vi "Calibration Routine(SubVI).vi"(10 "Calibrate":bool, 11 "File Path (Image Calibration 1)":path=path "\\\\hs2.lboro.ac.uk\\mmbc4/1_Univesity Work/Mechatronics/Machine Vision/Harry_Kane_Project/A3_table_cal_2.png") -> (0 "error out":errorcluster, 1 "Boolean":bool, 3 "Refnum out":T1(plugin-control))   [LabVIEW 2013]
uses:
  <vilib>/vision/driver/NI_Vision_Acquisition_Software.lvlib
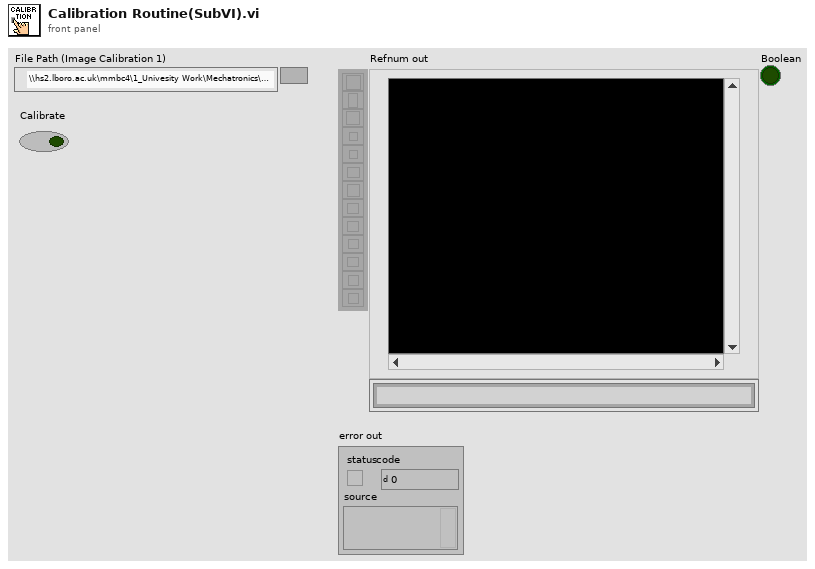
[diagram p1: front panel]
types:
  T1 = typedef "IMAQ Image.ctl" = refnum<image>
  T2 = typedef "Image Type" = u32
  T3 = typedef "IMAQdx.ctl" = refnum<k21>
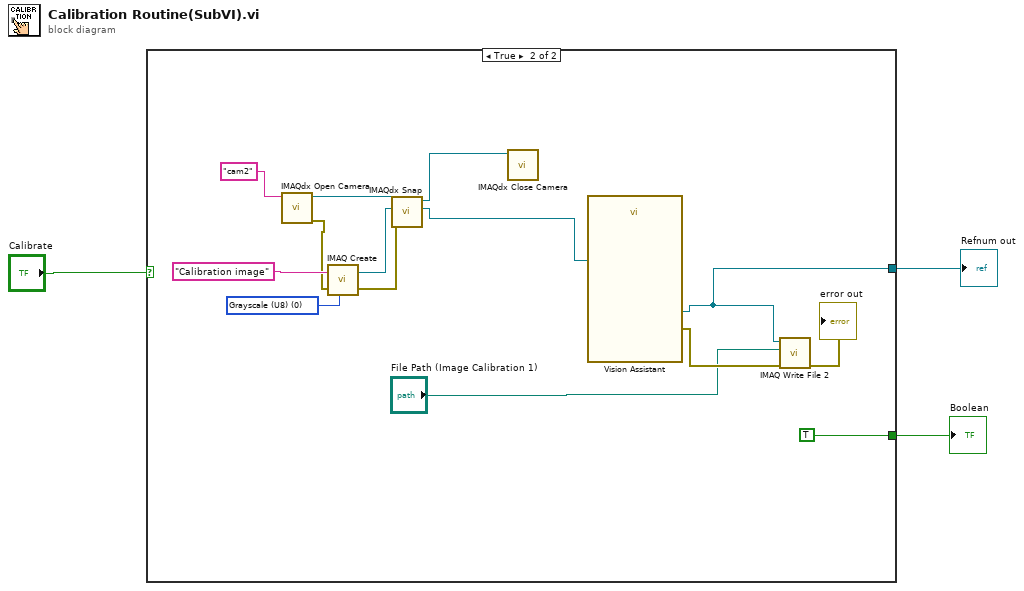
[diagram p0: block diagram]
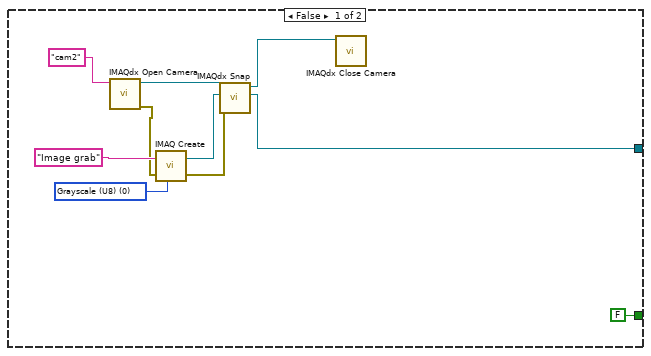
[diagram p2: hidden frame]
diagram:
  n1 = case shown="True" "Calibrate" {
    tunnel: [w5 w15] -> w3
    tunnel: [FALSE TRUE] -> w1
    frame False {
      w12 = T2 0 items=["Grayscale (U8)", "Grayscale (I16)", "Grayscale (SGL)", "Complex (CSG)", "RGB (U32)", "HSL (U32)", "RGB (U64)", "Grayscale (U16)"] ("Image Type")
      n2 = call <vilib>:"IMAQdx Open Camera.vi"("Session In"="cam2" ("Interface Name")) -> ("error out"=w6:errorcluster, "Session Out"=w7:T3)  [unwired: 9 in]
      n3 = call "IMAQ Create"("Image Name"="Image grab", "Image Type"=w12, "error in (no error)"=w6) -> ("New Image"=w11:T1, "error out"=w10:errorcluster)  [unwired: 2 in]
      n4 = call <vilib>:"IMAQdx Snap.vi"("error in"=w10, "Image In"=w11, "Session In"=w7) -> ("Image Out"=w5:T1, "Session Out"=w9:T3)  [unwired: 6 in, 1 out]
      n5 = call <vilib>:"IMAQdx Close Camera.vi"("Session In"=w9) -> ()  [unwired: 10 in, 1 out]
    }
    frame True {
      w26 = T2 0 items=["Grayscale (U8)", "Grayscale (I16)", "Grayscale (SGL)", "Complex (CSG)", "RGB (U32)", "HSL (U32)", "RGB (U64)", "Grayscale (U16)"] ("Image Type")
      n6 = call <vilib>:"IMAQdx Open Camera.vi"("Session In"="cam2" ("Interface Name")) -> ("error out"=w20:errorcluster, "Session Out"=w21:T3)  [unwired: 9 in]
      n7 = call "IMAQ Create"("Image Name"="Calibration image", "Image Type"=w26, "error in (no error)"=w20) -> ("New Image"=w25:T1, "error out"=w24:errorcluster)  [unwired: 2 in]
      n8 = call <vilib>:"IMAQdx Snap.vi"("error in"=w24, "Image In"=w25, "Session In"=w21) -> ("Image Out"=w19:T1, "Session Out"=w23:T3)  [unwired: 6 in, 1 out]
      n9 = call <vilib>:"IMAQdx Close Camera.vi"("Session In"=w23) -> ()  [unwired: 10 in, 1 out]
      n10 = call "Vision Assistant"("Image In"=w19) -> ("Image Out"=w15:T1, "error out"=w18:errorcluster)  [unwired: 25 in]
      n11 = call-poly "IMAQ Write File 2"("error in (no error)"=w18, "File Path"="File Path (Image Calibration 1)", "Image"=w15) -> ("error out"=→"error out":errorcluster)  [unwired: 7 in, 1 out]
    }
  }
  "Refnum out" <- w3
  "Boolean" <- w1
